vi "Abort.vi"(8 "error in (no error)":errorcluster, 11 "AbortManager in":refnum<class "AbortManager.lvclass">) -> (0 "error out":errorcluster, 3 "AbortManager out":refnum<class "AbortManager.lvclass">)   [LabVIEW 2020, in "Volatus.lvlib" / "AbortManager.lvclass"]
uses:
  AbortManager.lvclass
  AbortManager.lvclass/AbortManager.ctl
  AbortHandler Messages/Abort Msg/Abort Msg.lvclass
  <vilib>/ActorFramework/Message Enqueuer/Message Priority.ctl
  <vilib>/ActorFramework/Message Enqueuer/Message Enqueuer.lvclass
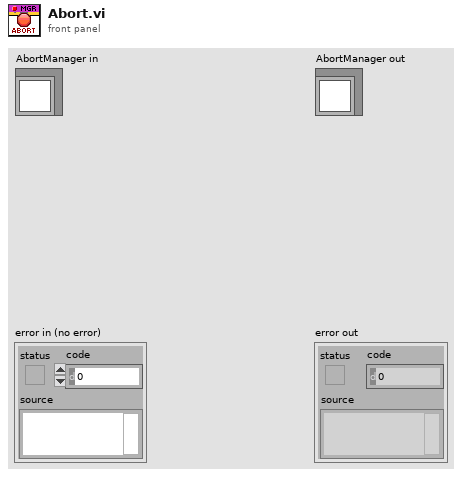
[diagram p1: front panel]
types:
  T1 = map{string, refnum<class "Message Enqueuer.lvclass">}
  T2 = typedef "Actor Framework.lvlib/Message Enqueuer.lvclass/Message Priority.ctl" = enum16{"Low", "Normal", "High"}
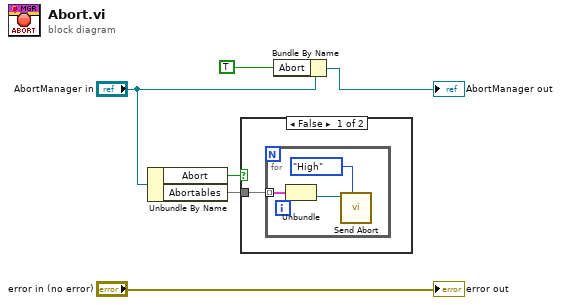
[diagram p0: block diagram]
diagram:
  n1 = Unbundle By Name("AbortManager in") -> ("Abort"=w1:bool, "Abortables"=w4:T1)
  n2 = case shown="False" w1 {
    tunnel: w4 -> [w7 _]
    frame False {
      n3 = for {
        tunnel: w7 -> [w10] mode=indexing
        n4 = Unbundle(w10) -> ("EnQr"=w9:refnum<class "Message Enqueuer.lvclass">)  [unwired: 1 out]
        n5 = call "Send Abort.vi"("Message Priority (Normal)"=Message_Priority."High", "Message Enqueuer"=w9) -> ()  [unwired: 8 in, 2 out]
      }
    }
    frame True {
    }
  }
  n6 = Bundle By Name(cluster="AbortManager in", "Abort"=TRUE) -> (→"AbortManager out":refnum<class "AbortManager.lvclass">)
  "error out" <- "error in (no error)"
